vi "OpenMCC.vi"(9 "Open":bool, 10 "Hardware Settings":T1={"Galvo Channels"="", "Detector Channels"="", "Galvo Trigger"="", "Shutter Lines"=[], "Max Acquisition Rate"=0.0, "Recommended Acquisition Rate"=0.0, "Galvo Write Rate"=0.0, "Max Timebase Frequency (Hz)"=0.0, "MCC Shutter Lines"=[], "Digital Image Multiplier"=0.0496, "Detector Task"="", "Shutter Tasks"=[], "Galvo Task"=""} {"Max Acquisition Rate" min=0.0 max=5000000.0 step=100000.0}, 11 "index":i32) -> (0 "error out":errorcluster)   [LabVIEW 2012]
uses:
  typedefs/HWsettings.ctl
  <vilib>/ULx/Create Channel.llb/ULx Create Channel (DO-Digital Output).vi
  <vilib>/ULx/Write.llb/ULx Write (Digital Bool 1Line 1Point).vi
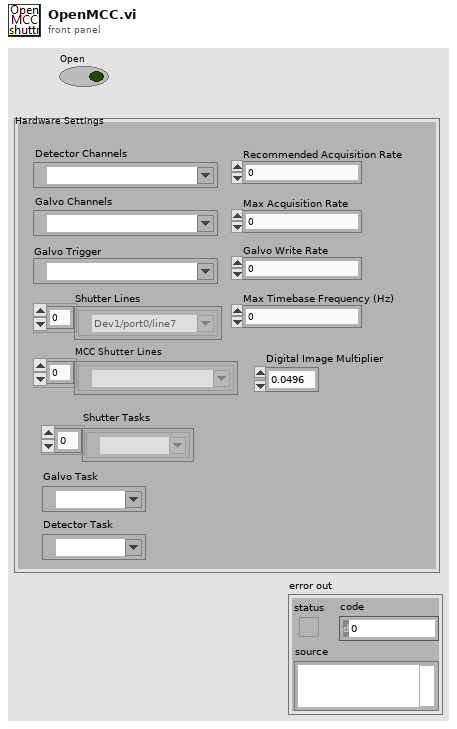
[diagram p1: front panel]
types:
  T1 = typedef "HWsettings.ctl" = cluster{"Galvo Channels":tag, "Detector Channels":tag, "Galvo Trigger":tag, "Shutter Lines":tag[], "Max Acquisition Rate":dbl, "Recommended Acquisition Rate":dbl, "Galvo Write Rate":dbl, "Max Timebase Frequency (Hz)":dbl, "MCC Shutter Lines":refnum<k21>[], "Digital Image Multiplier":dbl, "Detector Task":refnum<k21>, "Shutter Tasks":refnum<k21>[], "Galvo Task":refnum<k21>}
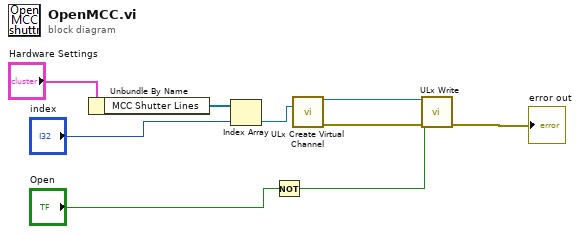
[diagram p0: block diagram]
diagram:
  n1 = Unbundle By Name("Hardware Settings") -> ("MCC Shutter Lines"=w7:refnum<k21>[])
  n2 = Index Array(array=w7, index="index") -> (element=w8:refnum<k21>)
  n3 = Not(x="Open") -> (.not. x?=w3:bool)
  n4 = call-poly <vilib>:"ULx Create Virtual Channel.vi"("lines"=w8) -> ("task out"=w6:refnum<k24>, "error out"=w2:errorcluster)  [unwired: 13 in]
  n5 = call-poly <vilib>:"ULx Write.vi"("task in"=w6, "data"=w3, "error in"=w2) -> ("error out"=→"error out":errorcluster)  [unwired: 10 in, 2 out]
